vi "HIL-Lab.vi"() -> ()   [LabVIEW 2018]
doc: "Simulator of heater model with PI controller, filter and datalogging"
uses:
  <vilib>/Simulation/Scripting/Companion Diagram/SimConfigNode/SimParams.ctl
  <vilib>/Simulation/Scripting/Companion Diagram/SimConfigNode/_simSolvers.ctl
  <vilib>/Simulation/Implementation/Shared/SIMSCR Execution Mode.ctl
  <vilib>/Simulation/Param Hierarchy/Typedefs/SIMPH Param Control Actions.ctl
  <vilib>/Simulation/Implementation/Shared/NILVSim_ParamChanged.vi
  <vilib>/Simulation/Implementation/Shared/NILVSIM_BeginStep.vi
  <vilib>/Simulation/Implementation/Shared/NILVSim_Manager.vi
  <vilib>/Utility/error.llb/Clear Errors.vi
  <vilib>/Simulation/Implementation/Shared/NILVSim_FinalizeModel.vi
  <vilib>/Simulation/Implementation/Shared/SIM Unbundle Sim Info.vi
  <vilib>/Simulation/Implementation/Shared/NILVSim_Initialize.vi
  <vilib>/Simulation/Utility/Implementation/NILVSim Get Time and IsAcceptedStep.vi
  <vilib>/Simulation/Implementation/Shared/SIMSH Read Queue.vi
  <vilib>/Simulation/Implementation/Shared/NILVSim_GetModelError.vi
  <vilib>/Simulation/Implementation/Shared/SIM Bundle Sim Info.vi
  <vilib>/Simulation/Implementation/XNodeFramework/SimXNode/SimX.xnode
  Example Code/Air Heater Black Box Model/Air Heater Black Box Model.vi
  <vilib>/Simulation/Scripting/Companion Diagram/SimConfigNode/SimDog.xnode
  Sim with delay.vi
  <vilib>/Simulation/Implementation/Shared/NI_SIM_Implementation.lvlib
panel:
  in  "stop":bool=TRUE
  out "Waveform Chart 2":dbl(graph)
  in  "Tab Control":T1(tab)
  in  "Temperature setpoint":dbl(knob)=20.0 scale=20.0..30.0
  in  "auto_man":bool
  in  "man_output u [V]":dbl
  out "u":dbl
  out "y":dbl=24.769142537907424
  in  "PID Parameters":T2={"Gain (Kp)"=1.57, "Integral Time (Ti, sec)"=16.0, "Derivative Time (Td, sec)"=0.0} {"Derivative Time (Td, sec)" format="%.3f"; "Integral Time (Ti, sec)" format="%.3f"; "Gain (Kp)" format="%.3f"}
  in  "Regulator Mode":string(combo)="Software PID"
  in  "Process Mode":string(combo)="Black Box"
  in  "Kh":dbl=3.5
  in  "theta_t":dbl=22.0
  in  "theta_d":dbl=2.0
  in  "T_env":dbl=21.0
  in  "Start_stop_file_writing":bool
  in  "Data file name:":path=path "C:/Users/haava/OneDrive/Master of Science/Control Engineering/Project/Prosjekt.lvm"
  in  "File header":string="%Logging of T_out vs reference and control signal.\n%Column 1: t [s]\n%Column 2: r [s]\n%Column 3: u [s]\n%Column 4: y [s]\n"
  out "Waveform Chart":cluster{"Tout [1-5V]":dbl, "T_out":dbl}(graph)
  # "Auto"
  # "Man"
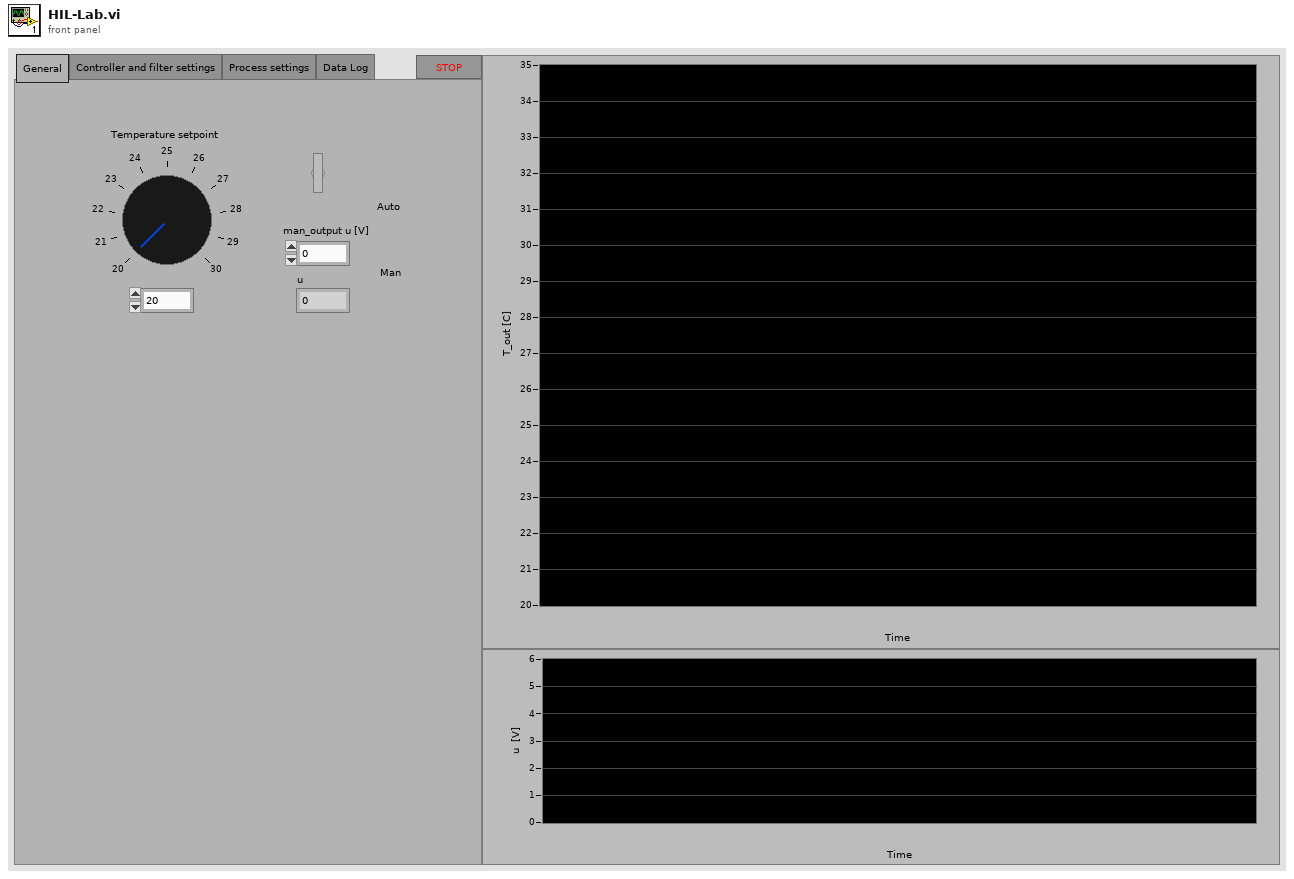
[diagram p1: front panel]
types:
  T1 = enum32{"General", "Controller and filter settings", "Process settings", "Data Log"}
  T2 = cluster{"Gain (Kp)":dbl, "Integral Time (Ti, sec)":dbl, "Derivative Time (Td, sec)":dbl}
  T3 = enum16{"Simulate to Completion", "Single Time-Step Simulation (Fixed Step Only)"}
  T4 = typedef "SIMSCR Execution Mode.ctl" = enum16{"Simulate to Completion", "Single Time-Step Simulation (Fixed Step Only)"}
  T5 = typedef "SIMPH Param Control Actions.ctl" = enum16{"get params", "set params"}
  T6 = cluster{"SIMSH Sim Time":dbl, "Select":cluster{"s? t:f":dbl}, "Linear Scaling with Points.vi":cluster{"y":dbl}, "Summation 3":cluster{"Result":dbl}, "Square Root":cluster{"sqrt(x)":dbl}, "Gaussian White Noise PtByPt.vi":cluster{"Gaussian white noise":dbl}, "Integrator":cluster{"output":dbl}, "Multiplication":cluster{"Result":dbl}, "Summation":cluster{"Result":dbl}, "Multiplication 2":cluster{"Result":dbl}, "Transport Delay":cluster{"output":dbl}, "Summation 2":cluster{"Result":dbl}}
  T7 = typedef "SimParams.ctl" = cluster{"Initial Time (s)":dbl, "Final Time (s)":dbl, "Step Size (s)":dbl, "ODE Solver":T8, "Minimum Step Size (s)":dbl, "Maximum Step Size (s)":dbl, "Relative Tolerance":dbl, "Absolute Tolerance":dbl, "Software Timing":bool, "Initial Step Size (s)":dbl, "Automatic Fixed Step Size?":bool, "Automatic Discrete Step Size?":bool, "Discrete Step Size (s)":dbl, "Calculate using Time Step":bool, "Solver Wired?":bool, "Prev.Frm.Expected End":u64, "Prev.Frm.Actual End":u64, "Prev.Frm.Finished Late?":bool, "Prev.Iter.Expected End":u64, "Prev.Iter.Actual End":u64, "Prev.Iter.Finished Late?":bool, "Expected Iteration Start":u64, "Actual Iteration Start":u64, "Expected Frame Start":u64, "Actual Frame Start":u64, "Source Name":string, "Name":string, "Period":i64, "Deadline":i64, "Offset":i64, "Start":i64, "Priority":i32, "Timeout":i32, "Processor":i32, "Mode":enum32{"No Change", "Process missed periods, maintain original phase", "Discard missed periods, maintain original phase", "Process missed periods, ignore original phase", "Discard missed periods, ignore original phase"}, "Wakeup reason":enum32{"Normal", "Aborted", "Asynchronous wakeup", "Timing source error", "Timed loop error", "Timeout"}, "Error":errorcluster, "Source Type":string, "Secondary Source Type":string, "Global End Time":u64, "Global Start Time":u64, "Full Solver Reset":bool, "Execution Mode":T4, "Nan/Inf Check":bool, "Custom Solver Library":string, "Solver Is Variable":bool, "custom solver name":string, "Signal Collection Decimation":u32}
  T8 = typedef "_simSolvers.ctl" = enum16{"Runge-Kutta 1 (Euler)", "Runge-Kutta 2", "Runge-Kutta 3", "Runge-Kutta 4", "Runge-Kutta 23 (variable)", "Runge-Kutta 45 (variable)", "BDF (variable)", "Adams-Moulton (variable)", "Rosenbrock (variable)", "Discrete States Only", "SDIRK 4 (variable)", "Radau 5 (variable)", "Radau 9 (variable)", "Radau 13 (variable)", "Radau [Variable Order] (variable)", "Gear's Method (variable)", "Linearizer", "State Query", "Trim Eval", "Custom Solver"}
  T9 = cluster{"SIMSH Sim Time":dbl, "upper limit":dbl, "Integrator":cluster{"output":dbl}, "Multiplication 2":cluster{"Result":dbl}, "Summation 2":cluster{"Result":dbl}, "Summation":cluster{"Result":dbl}, "Multiplication":cluster{"Result":dbl}, "Transport Delay":cluster{"output":dbl}}
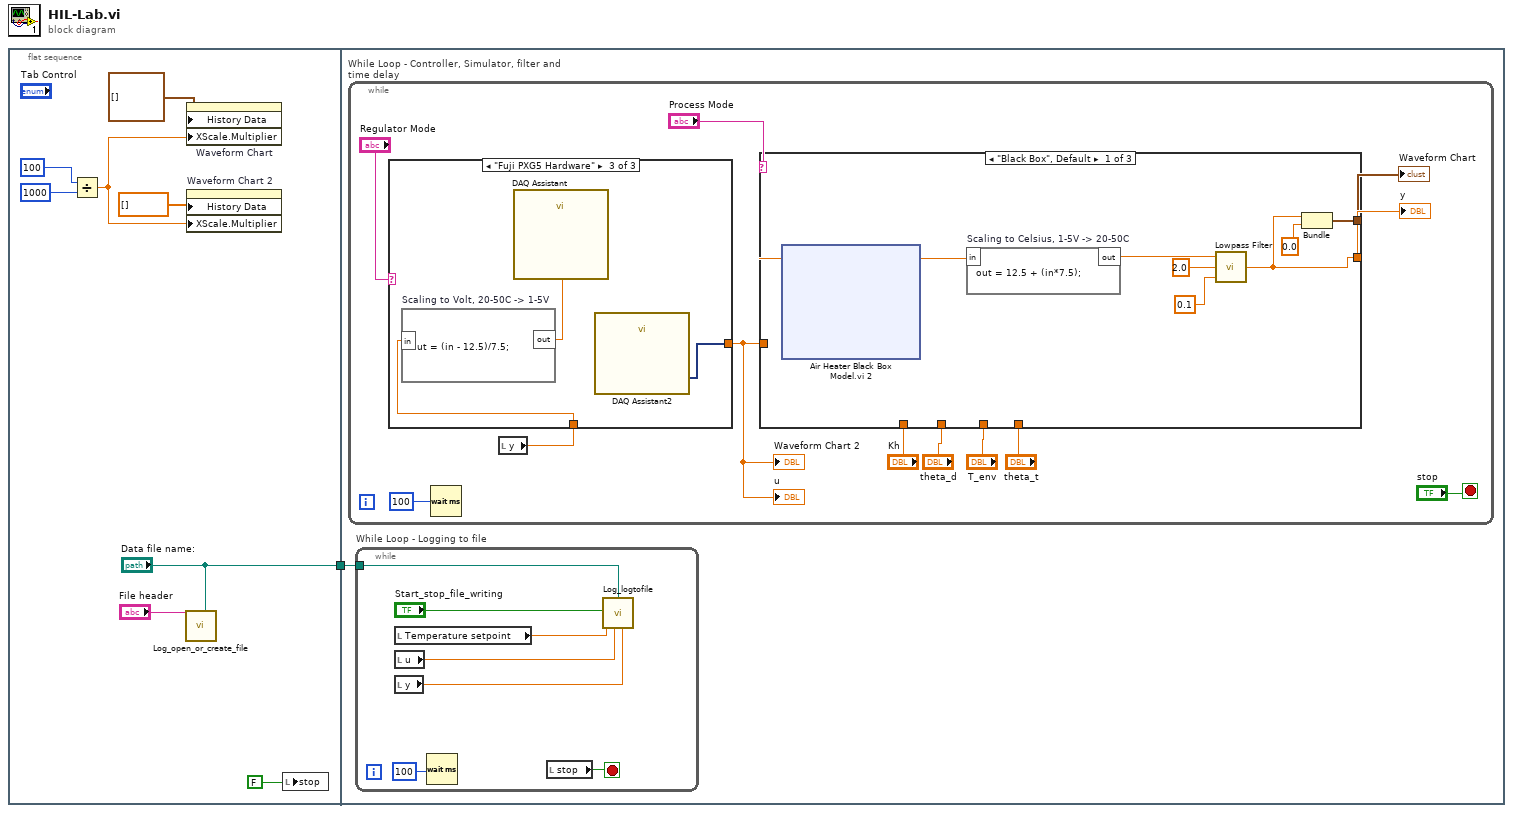
[diagram p0: block diagram]
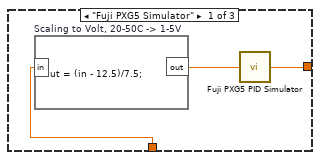
[diagram p2: hidden frame]
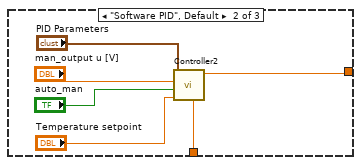
[diagram p3: hidden frame]
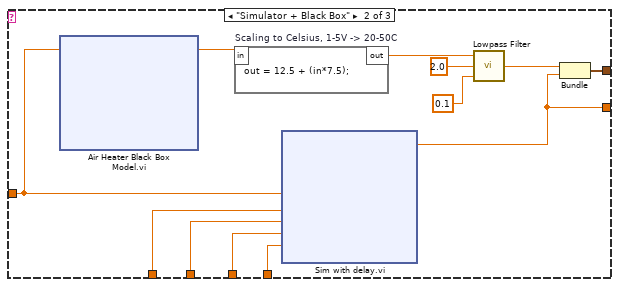
[diagram p4: hidden frame]
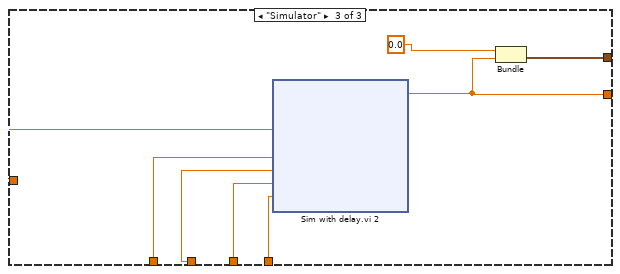
[diagram p5: hidden frame]
diagram:
  n1 = flat-sequence {
    tunnel: ["Data file name:"] -> w1
    tunnel: w1 -> [w10]
    frame #0 {
      n2 = Divide(x=u32 100 ("milliseconds to wait"), y=u32 1000 ("x")) -> (x/y=w6:dbl)
      n3 = call "Log_open_or_create_file.vi"("Data file name:"="Data file name:", "File header"="File header") -> ()  [unwired: 10 in]
      n4 = property on="Waveform Chart" class="WFChart (strict)"("History Data"=cluster{"Tout [1-5V]":dbl, "T_out":dbl}[] [], "XScale.Multiplier"=w6) -> ()  [unwired: 2 in, 2 out]
      n5 = property on="Waveform Chart 2" class="WFChart (strict)"("History Data"=dbl[] [], "XScale.Multiplier"=w6) -> ()  [unwired: 2 in, 2 out]
      n6 = local write "stop"(FALSE ("stop")) -> ()
    }
    frame #1 {
      n7 = while "While Loop - Controller, Simulator, filter and time delay" {
        stop <- "stop" stop-if-true
        n8 = Wait (ms)(milliseconds to wait=u32 100) -> ()  [unwired: 1 out]
        n9 = local read "y"() -> (w25:dbl)
        n10 = case shown="\"Fuji PXG5 Hardware\"" "Regulator Mode" {
          tunnel: [w31 w36 w39] -> w26
          tunnel: w25 -> [w32 w34 w41]
          frame "Fuji PXG5 Simulator" {
            n11 = formula code="out = (in - 12.5)/7.5;" "Scaling to Volt, 20-50C -> 1-5V"("in"=w32) -> ("out"=w30:dbl)
            n12 = call "Fuji PXG5 PID Simulator.vi"("Input (1-5V)"=w30) -> ("Output (0-5V)"=w31:dbl)
          }
          frame "Software PID", Default {
            n13 = call "Controller2.vi"("process variable"=w34, "setpoint"="Temperature setpoint", "auto_man"="auto_man", "man_output u [V]"="man_output u [V]", "PID gains"="PID Parameters") -> ("output"=w36:dbl)  [unwired: 6 in]
          }
          frame "Fuji PXG5 Hardware" {
            n14 = formula code="out = (in - 12.5)/7.5;" "Scaling to Volt, 20-50C -> 1-5V"("in"=w41) -> ("out"=w40:dbl)
            n15 = call "DAQ Assistant"("data"=w40) -> ()  [unwired: 17 in, 2 out]
            n16 = call "DAQ Assistant2"() -> ("data"=w39:dynamicdata)  [unwired: 17 in, 2 out]
          }
        }
        "Waveform Chart 2" <- w26
        "u" <- w26
        n17 = case shown="\"Black Box\", Default" "Process Mode" {
          tunnel: [w42 w305 w823] -> w27
          tunnel: w26 -> [w46 w295 w822]
          tunnel: [w44 w300 w825] -> w24
          tunnel: "Kh" -> [_ w299 w821]
          tunnel: "T_env" -> [_ w298 w819]
          tunnel: "theta_d" -> [_ w297 w820]
          tunnel: "theta_t" -> [_ w296 w818]
          frame "Black Box", Default {
            n18 = xnode "Air Heater Black Box Model.vi 2"("Control Signal [0-5V]"=w46) -> ("Tout [1-5V]"=w45:dbl)  [unwired: 2 in, 1 out]
            n19 = formula code="out = 12.5 + (in*7.5);" "Scaling to Celsius, 1-5V -> 20-50C"("in"=w45) -> ("out"=w49:dbl)
            n20 = call "Lowpass Filter.vi"("Ts [s]"=0.1, "Tf [s]"=2.0, "Filter Input"=w49) -> ("Filter Output"=w42:dbl)
            n21 = Bundle("Filter Output"=w42, "Tf [s]"=0.0) -> (w44:cluster{"Filter Output":dbl, "Tf [s]":dbl})  [unwired: 1 in]
          }
          frame "Simulator + Black Box" {
            n22 = xnode "Air Heater Black Box Model.vi"("Control Signal [0-5V]"=w295) -> ("Tout [1-5V]"=w306:dbl)  [unwired: 2 in, 1 out]
            n23 = formula code="out = 12.5 + (in*7.5);" "Scaling to Celsius, 1-5V -> 20-50C"("in"=w306) -> ("out"=w304:dbl)
            n24 = xnode "Sim with delay.vi"("T_env"=w298, "theta_d"=w297, "theta_t"=w296, "Kh"=w299, "u"=w295) -> ("T_out"=w305:dbl)  [unwired: 2 in, 7 out]
            n25 = call "Lowpass Filter.vi"("Ts [s]"=0.1, "Tf [s]"=2.0, "Filter Input"=w304) -> ("Filter Output"=w301:dbl)
            n26 = Bundle("Filter Output"=w301, "T_out"=w305) -> (w300:cluster{"Filter Output":dbl, "T_out":dbl})  [unwired: 1 in]
          }
          frame "Simulator" {
            n27 = xnode "Sim with delay.vi 2"("T_env"=w819, "theta_d"=w820, "theta_t"=w818, "Kh"=w821, "u"=w822) -> ("T_out"=w823:dbl)  [unwired: 2 in, 7 out]
            n28 = Bundle("T_env"=0.0, "T_out"=w823) -> (w825:cluster{"T_env":dbl, "T_out":dbl})  [unwired: 1 in]
          }
        }
        "Waveform Chart" <- w24
        "y" <- w27
      }
      n29 = while "While Loop - Logging to file" {
        tunnel: w10 -> [w11]
        stop <- w12 stop-if-true
        n30 = local read "Temperature setpoint"() -> (w16:dbl)
        n31 = local read "u"() -> (w15:dbl)
        n32 = local read "y"() -> (w13:dbl)
        n33 = Wait (ms)(milliseconds to wait=u32 100 ("sample time")) -> ()  [unwired: 1 out]
        n34 = local read "stop"() -> (w12:bool)
        n35 = call "Log_logtofile.vi"("Waveform Chart in"=w15, "y"=w13, "Temperature setpoint"=w16, "Start_stop_file_writing"="Start_stop_file_writing", "Data file name:"=w11) -> ()  [unwired: 7 in]
      }
    }
  }
